vi "DUAL GAUGE-Range extension.vi"(7 "W/R":bool, 8 "Fehler (Eingang)":errorcluster, 9 "Gauge CH 2":i32(ring) items=["range extension off", "range extension on"], 10 "Gauge CH 1":i32(ring) items=["range extension off", "range extension on"], 11 "Referenz in":refnum<visa-resource-name>) -> (0 "Cluster (Ausgang)":errorcluster, 1 "Gauge CH 2 out":i32(ring) items=["range extension off", "range extension on"], 2 "Gauge CH 1 out":i32(ring) items=["range extension off", "range extension on"], 3 "Referenz out":refnum<visa-resource-name>)   [LabVIEW 2013, in "Dual Gauge.lvlib"]
uses:
  Dual Gauge.lvlib
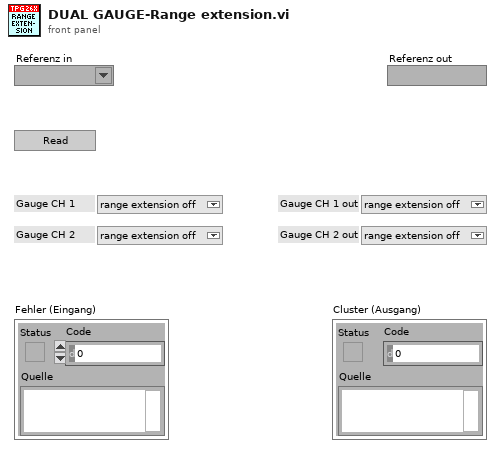
[diagram p1: front panel]
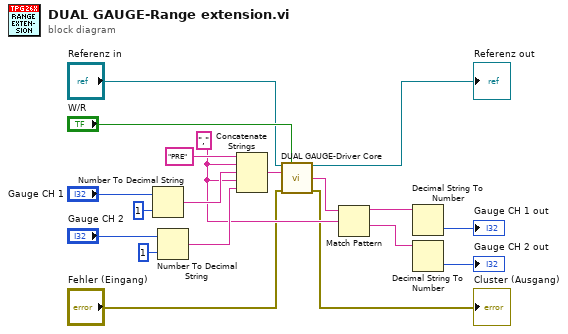
[diagram p0: block diagram]
diagram:
  w9 = "," ("Command")
  n1 = Number To Decimal String(number="Gauge CH 1", width (-)=i16 1) -> (decimal integer string=w12:string)
  n2 = Number To Decimal String(number="Gauge CH 2", width (-)=i16 1) -> (decimal integer string=w11:string)
  n3 = Concatenate Strings("PRE" ("Command"), w9, w12, w9, w11) -> (w5:string)
  n4 = call "DUAL GAUGE-Driver Core.vi"("Referenz in"="Referenz in", "Write/Read"="W/R", "Command"=w5, "Fehler (Eingang)"="Fehler (Eingang)") -> ("Referenz out"=→"Referenz out":refnum<visa-resource-name>, "String Out"=w10:string, "Cluster (Ausgang)"=→"Cluster (Ausgang)":errorcluster)  [unwired: 9 in]
  n5 = Match Pattern(string=w10, regular expression=w9) -> (before substring=w8:string, after substring=w6:string)  [unwired: 1 in, 2 out]
  n6 = Decimal String To Number(string=w8) -> (number=→"Gauge CH 1 out":i32)  [unwired: 2 in, 1 out]
  n7 = Decimal String To Number(string=w6) -> (number=→"Gauge CH 2 out":i32)  [unwired: 2 in, 1 out]
